vi "Analog Mapping Query.vi"(8 "error in (no error)":errorcluster, 11 "Refnum In":refnum<vi>) -> (0 "error out":errorcluster, 2 "Board Capabilities":map{i32, T1}(c390), 3 "Refnum Out":refnum<vi>)   [LabVIEW 2020]
doc: "VI that will request the analog mapping of pins, i.e. which pins are A0, A1, A2,..."
uses:
  Controls/FirmataPinCapabilitiesAndAnalogMapping.ctl
  Controls/FirmataPinCapability.ctl
  FirmataClient.v1/controls/FirmataPinModes.ctl
  FirmataClient.v1/FirmataClient.lvlib
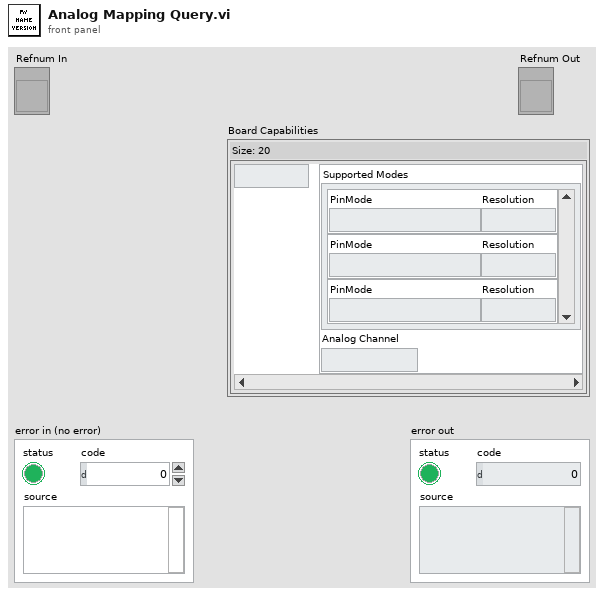
[diagram p1: front panel]
types:
  T1 = typedef "FirmataPinCapabilitiesAndAnalogMapping.ctl" = cluster{"Supported Modes":T2[], "Analog Channel":u8}
  T2 = typedef "FirmataPinCapability.ctl" = cluster{"PinMode":T3, "Resolution":u8}
  T3 = typedef "FirmataClient.lvlib/FirmataPinModes.ctl" = enum16{"DigitalInput", "DigitalOutput", "AnalogInput", "PWM", "Servo", "Shift", "I2C", "OneWire", "Stepper", "Encoder", "Serial", "InputPullup", "Extended.SPI", "Extended.Sonar", "Extended.Tone", "Extended.DHT"}
  T4 = typedef "FirmataProtocolConstants.ctl" = u16
  T5 = typedef "Parameters.ctl" = cluster{"Transport Parameters":T6, "Board Capabilities":map{i32, T1}}
  T6 = typedef "TransportParameters.ctl" = cluster{"Serial Communication":cluster{"Comport":refnum<visa-resource-name>, "No Response Timeout Ms":u32, "Response Complete Timeout Ms":u32, "Max Rx Length":u32, "Baud Rate":u32}, "Selected Transport":T7, "Initializer File Path":path, "Cleaner File Path":path, "Transporter File Path":path}
  T7 = typedef "SupportedTransports.ctl" = enum16{"Serial Communication Port"}
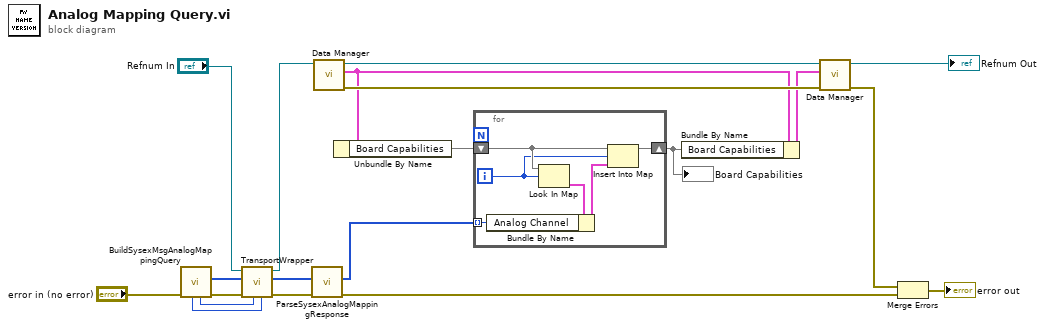
[diagram p0: block diagram]
diagram:
  n1 = call "BuildSysexMsgAnalogMappingQuery.vi"("error in"="error in (no error)") -> ("error out"=w20:errorcluster, "GetAnalogMappingMessage"=w15:u8[], "ReplyFirstByte"=w17:T4, "ReplyLength"=w16:i32)  [unwired: 7 in]
  n2 = call "TransportWrapper.vi"("ReplyLength"=w16, "ReplyFirstByte"=w17, "error in"=w20, "Message In"=w15, "Refnum In"="Refnum In") -> ("error out"=w14:errorcluster, "Message Out"=w5:u8[], "Refnum Out"=w13:refnum<vi>)  [unwired: 4 in]
  n3 = call "ParseSysexAnalogMappingResponse.vi"("error in"=w14, "Sysex Message"=w5) -> ("error out"=w8:errorcluster, "AnalogChannels"=w1:u8[])  [unwired: 7 in, 1 out]
  n4 = call "Data Manager.vi"("Refnum In"=w13) -> ("error out"=w10:errorcluster, "Data Out"=w4:T5, "Refnum Out"=w12:refnum<vi>)  [unwired: 8 in]
  n5 = Unbundle By Name(w4) -> ("Board Capabilities"=w2:map{i32, T1})
  n6 = for {
    shift-right: [w26] -> w3
    shift-left: w2 -> [w25]
    tunnel: w1 -> [w22] mode=indexing
    i -> [w21]
    n7 = Look In Map(map=w25, key=w21) -> (value=w24:T1)  [unwired: 1 in, 1 out]
    n8 = Bundle By Name(cluster=w24, "Analog Channel"=w22) -> (w23:T1)
    n9 = Insert Into Map(map in=w25, key=w21, value=w23) -> (map out=w26:map{i32, T1})  [unwired: 2 out]
  }
  "Board Capabilities" <- w3
  n10 = Bundle By Name(cluster=w4, "Board Capabilities"=w3) -> (w6:T5)
  n11 = call "Data Manager.vi"("error in (no error)"=w10, "Data In"=w6, "Refnum In"=w12) -> ("error out"=w9:errorcluster, "Refnum Out"=→"Refnum Out":refnum<vi>)  [unwired: 6 in, 1 out]
  n12 = Merge Errors(w9, w8) -> (→"error out":errorcluster)
